vi "Unflatten from MessageString.vi"(8 "error in (no error)":errorcluster, 11 "Msg String":T2={"Flatten Msg"="", "Message Priority"=enum."Normal"}) -> (0 "error out":errorcluster, 2 "Message Priority":T1=enum."Normal", 3 "Actor Framework:Message":refnum<class "Message.lvclass">)   [LabVIEW 2014, in "Network Stream.lvlib" / "Network Stream.lvclass"]
uses:
  Network Stream.lvclass
  MessageString.ctl
  <vilib>/ActorFramework/Message Enqueuer/Message Priority.ctl
  <vilib>/ActorFramework/Message/Message.lvclass
  <vilib>/ActorFramework/Message Enqueuer/Message Enqueuer.lvclass
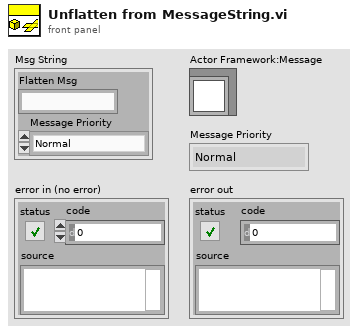
[diagram p1: front panel]
types:
  T1 = typedef "Actor Framework.lvlib/Message Enqueuer.lvclass/Message Priority.ctl" = enum16{"Low", "Normal", "High"}
  T2 = typedef "Network Stream.lvlib/Network Stream.lvclass/MessageString.ctl" = cluster{"Flatten Msg":string, "Message Priority":T1}
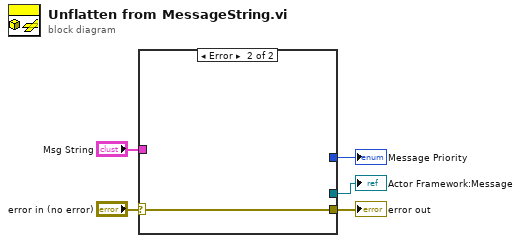
[diagram p0: block diagram]
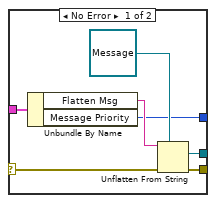
[diagram p2: hidden frame]
diagram:
  n1 = case shown="Error" "error in (no error)" {
    selector: "error in (no error)" -> [w9 w13]
    tunnel: [w8 w13] -> w5
    tunnel: "Msg String" -> [w12 _]
    tunnel: [w7 _] -> w2
    tunnel: [w6 _] -> w1
    frame No Error {
      n2 = Unbundle By Name(w12) -> ("Flatten Msg"=w10:string, "Message Priority"=w6:T1)
      n3 = Unflatten From String(type=refnum<class "Message.lvclass"> refnum ("Actor Framework.lvlib:Message.lvclass"), binary string=w10, error in (no error)=w9) -> (value=w7:refnum<class "Message.lvclass">, error out=w8:errorcluster)  [unwired: 2 in, 1 out]
    }
    frame Error {
    }
  }
  "Actor Framework:Message" <- w2
  "error out" <- w5
  "Message Priority" <- w1
